vi "CallOutputList.vi"(5 "list":string, 9 "SubVI in":refnum<class "SubVI.lvclass">) -> (3 "SubVI out":refnum<class "SubVI.lvclass">, 4 "call outputs":string)   [LabVIEW 2014, in "Raspberry Pi Compatible Compiler for LabVIEW.lvlib" / "SubVI.lvclass"]
uses:
  SubVI.lvclass
  Python/Parsing/ListTypesTD.ctl
  Node/Node.lvclass
  Terminal/Terminal.lvclass
  Python/Parsing/Python Functions.lvlib
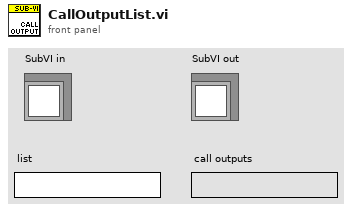
[diagram p1: front panel]
types:
  T1 = typedef "Raspberry Pi Compatible Compiler for LabVIEW.lvlib/Python Functions.lvlib/ListTypesTD.ctl" = enum16{"list", "tuple", "parameter list", "output list", "return values"}
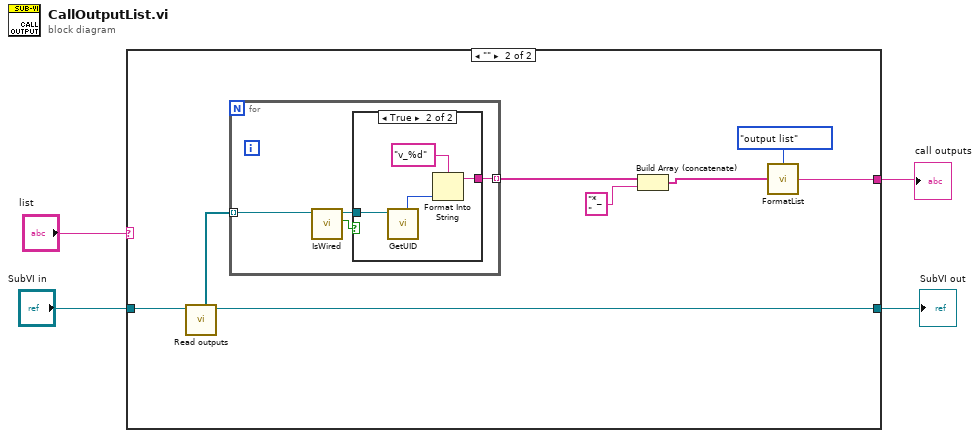
[diagram p0: block diagram]
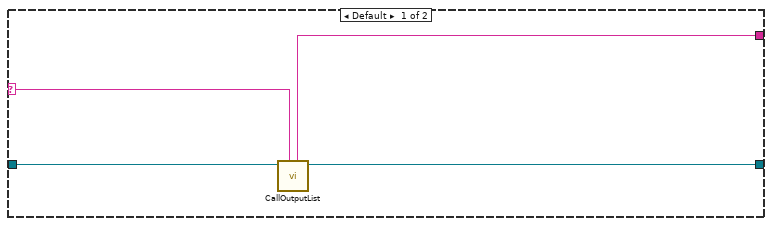
[diagram p2: hidden frame]
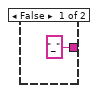
[diagram p3: hidden frame]
diagram:
  n1 = case shown="\"\"" "list" {
    selector: "list" -> [w7 _]
    tunnel: "SubVI in" -> [w8 w14]
    tunnel: [w6 w13] -> w3
    tunnel: [w5 w12] -> w2
    frame Default {
      n2 = call-parent "CallOutputList.vi"("list"=w7, "Node in"=w8) -> ("Node out"=w5:refnum<class "SubVI.lvclass">, "call outputs"=w6:string)  [unwired: 6 in]
    }
    frame "" {
      n3 = call-dynamic "Read outputs.vi"("Node in"=w14) -> ("Node out"=w12:refnum<class "SubVI.lvclass">, "outputs"=w16:refnum<class "Terminal.lvclass">[])  [unwired: 7 in]
      n4 = for {
        tunnel: w16 -> [w17] mode=indexing
        tunnel: [w20] -> w11 mode=indexing
        n5 = call "IsWired.vi"("Terminal in"=w17) -> ("wired"=w18:bool, "Terminal out"=w19:refnum<class "Terminal.lvclass">)  [unwired: 6 in, 1 out]
        n6 = case shown="True" w18 {
          tunnel: ["_" w25] -> w20
          tunnel: w19 -> [_ w23]
          frame False {
          }
          frame True {
            n7 = call-dynamic "GetUID.vi"("GObject in"=w23) -> ("UID"=w22:i32)  [unwired: 6 in, 2 out]
            n8 = Format Into String(format string="v_%d", w22) -> (resulting string=w25:string)  [unwired: 2 in, 1 out]
          }
        }
      }
      n9 = Build Array (concatenate)(w11, "*_") -> (w9:string[])
      n10 = call "FormatList.vi"("values"=w9, "type"=ListTypesTD."output list") -> ("python object"=w13:string)
    }
  }
  "call outputs" <- w3
  "SubVI out" <- w2
